vi "Write Bank Type.vi"(9 "Bank Type":T1, 11 "Bank in":refnum<class "Bank.lvclass">) -> (3 "Bank out":refnum<class "Bank.lvclass">)   [LabVIEW 2019, in "LRUTS FPGA IP.lvlib" / "Bank.lvclass"]
uses:
  Bank.lvclass
  Bank Type.ctl
  Bank.lvclass/Bank.ctl
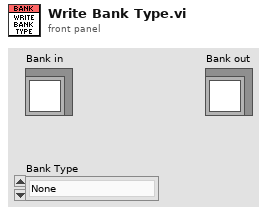
[diagram p1: front panel]
types:
  T1 = typedef "LRUTS FPGA IP.lvlib/Bank.lvclass/Bank Type.ctl" = enum16{"None", "Discrete Acquisition", "Discrete Generation", "PWM Acquisition", "PWM Generation"}
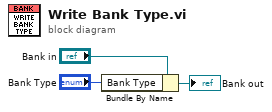
[diagram p0: block diagram]
diagram:
  n1 = Bundle By Name(cluster="Bank in", "Bank Type"="Bank Type") -> (→"Bank out":refnum<class "Bank.lvclass">)
